vi "SCLN_ServerNewID.vi"(3 "Server Port":i32, 4 "Listener ID IN":refnum<k5>) -> (1 "Listener ID OUT":refnum<k5>)   [LabVIEW 2015]
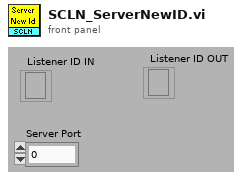
[diagram p1: front panel]
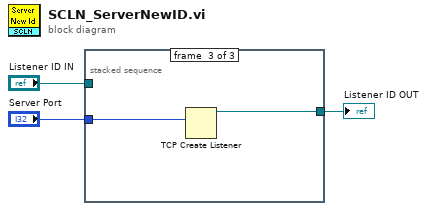
[diagram p0: block diagram]
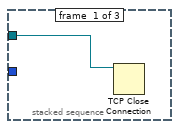
[diagram p2: hidden frame]
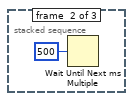
[diagram p3: hidden frame]
diagram:
  n1 = stacked-sequence {
    tunnel: [_ _ w7] -> w3
    tunnel: "Server Port" -> [_ _ w6]
    tunnel: "Listener ID IN" -> [w4 _ _]
    frame #0 {
      n2 = TCP Close Connection(connection ID=w4) -> ()  [unwired: 2 in, 2 out]
    }
    frame #1 {
      n3 = Wait Until Next ms Multiple(millisecond multiple=500) -> ()  [unwired: 1 out]
    }
    frame #2 {
      n4 = TCP Create Listener(10:w6) -> (3:w7:refnum<k5>)  [unwired: 4 in, 2 out]
    }
  }
  "Listener ID OUT" <- w3
